vi "Format List Results String.vi"(3 "Items (0)":i32, 4 "Plural Items (\"Items\")":string="Items", 5 "Singular Item (\"Item\")":string="Item") -> (2 "Result String":string)   [LabVIEW 2011]
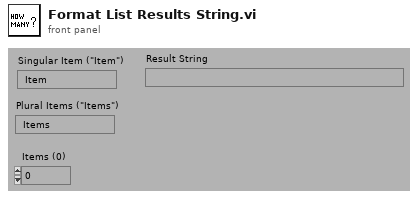
[diagram p1: front panel]
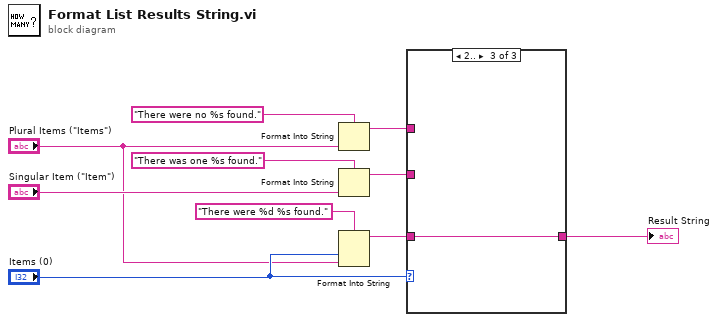
[diagram p0: block diagram]
diagram:
  n1 = Format Into String(format string="There were no %s found." ("search string"), "Plural Items (\"Items\")") -> (resulting string=w6:string)  [unwired: 2 in, 1 out]
  n2 = Format Into String(format string="There was one %s found." ("search string"), "Singular Item (\"Item\")") -> (resulting string=w2:string)  [unwired: 2 in, 1 out]
  n3 = Format Into String(format string="There were %d %s found." ("search string"), "Items (0)", "Plural Items (\"Items\")") -> (resulting string=w10:string)  [unwired: 2 in, 1 out]
  n4 = case shown="2.." "Items (0)" {
    tunnel: w2 -> [_ w12 _]
    tunnel: w10 -> [_ _ w13]
    tunnel: [w11 w12 w13] -> w8
    tunnel: w6 -> [w11 _ _]
    frame 0, Default {
    }
    frame 1 {
    }
    frame 2.. {
    }
  }
  "Result String" <- w8
